vi "GetStartingMainViReference.vi"(8 "error in (no error)":errorcluster caption="Fehler (Eingang, kein Fehler)", 11 "ApplicationInititialisation Eingang":refnum<class "ApplicationInititialisation.lvclass"> caption="DNL_LabVIEW Object in") -> (0 "error out":errorcluster caption="Fehler (Ausgang)", 1 "String":string, 2 "vi reference":refnum<vi>, 3 "ApplicationInititialisation Ausgang":refnum<class "ApplicationInititialisation.lvclass"> caption="DNL_LabVIEW Object out")   [LabVIEW 2013, in "ApplicationInititialisation.lvclass"]
uses:
  ApplicationInititialisation.lvclass
panel:
  out "Array":string[](array[string])
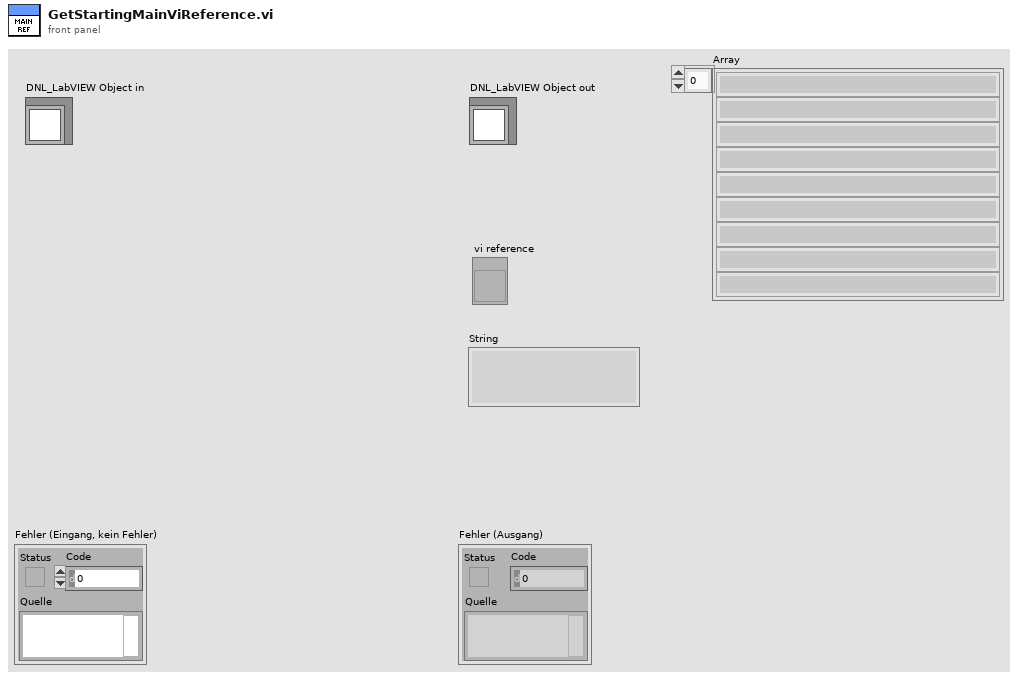
[diagram p1: front panel]
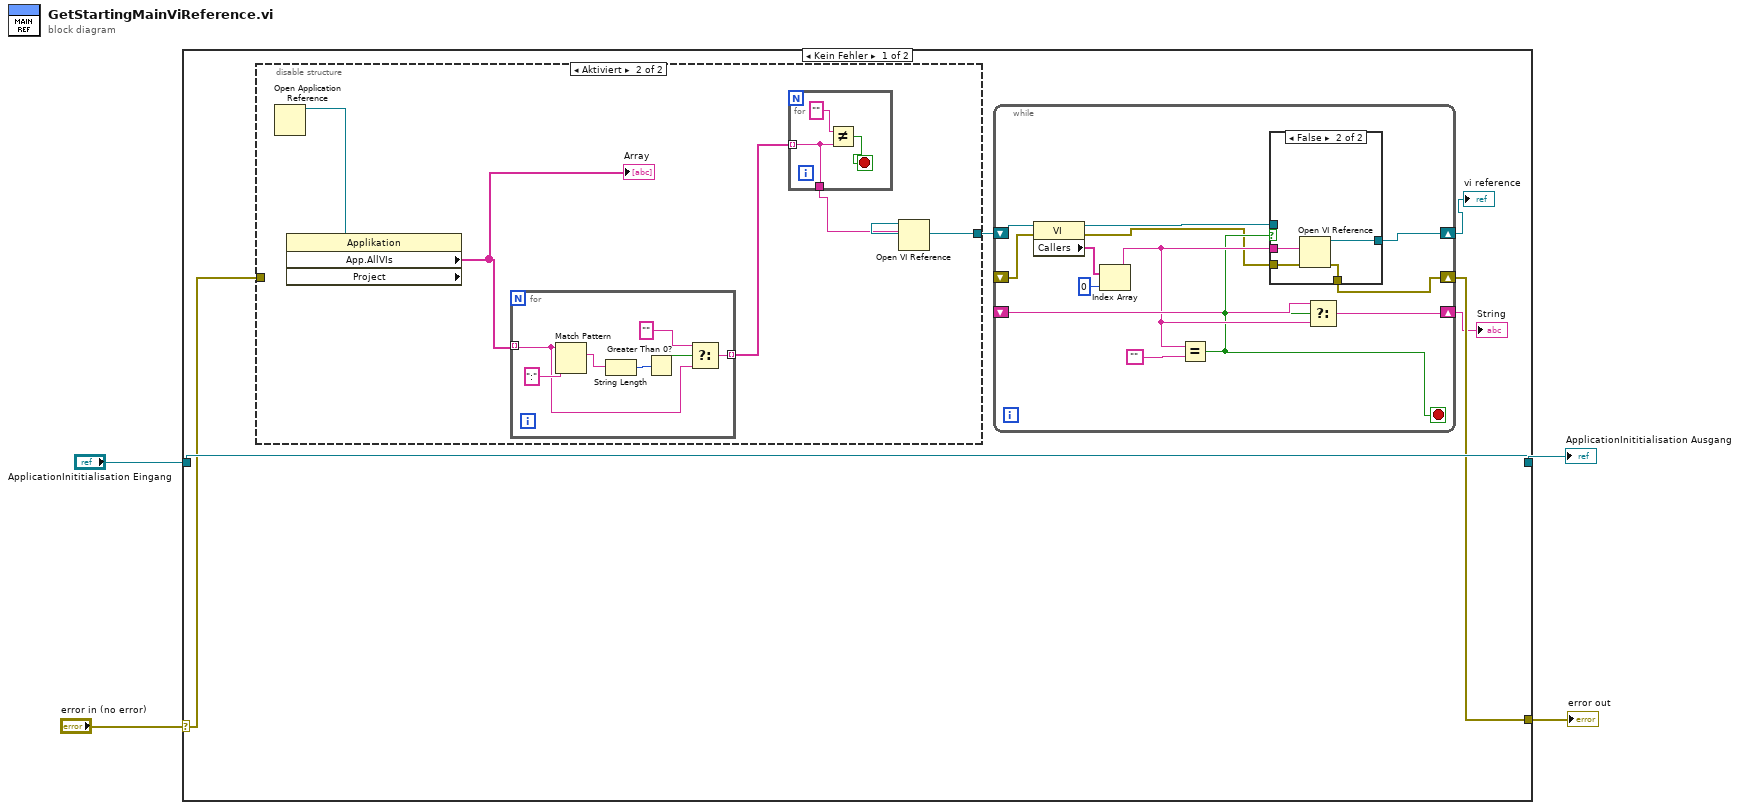
[diagram p0: block diagram]
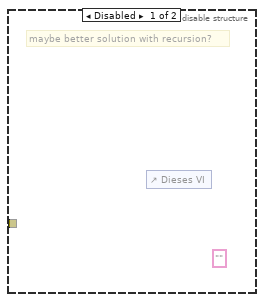
[diagram p3: hidden frame]
diagram:
  n1 = case shown="Kein Fehler" "error in (no error)" {
    selector: "error in (no error)" -> [w9 w47]
    tunnel: [w10 w48] -> w2
    tunnel: "ApplicationInititialisation Eingang" -> [w10 w48]
    tunnel: [w6 w47] -> w1
    frame No Error {
      n2 = disable-structure shown="Aktiviert" {
        disable-tunnel: [_ w35] -> w8
        disable-tunnel: w9 -> [w30 _]
        frame Disabled {
          (unwired) ""
          # "maybe better solution with recursion?"
          n3 = control-ref of="Dieses VI"() -> (w31:refnum<vi>)
        }
        frame Enabled {
          n4 = Open Application Reference() -> (3:w36:refnum<vi>)  [unwired: 4 in, 1 out]
          n5 = property class="Applikation" props=["App.AllVIs", "Project"](reference=w36) -> ("App.AllVIs"=w32:string[])  [unwired: 1 in, 3 out]
          "Array" <- w32
          n6 = for {
            tunnel: w32 -> [w41] mode=indexing
            tunnel: [w40] -> w34 mode=indexing
            n7 = Match Pattern(string=w41, regular expression=":" ("Format-String")) -> (match substring=w43:string)  [unwired: 1 in, 3 out]
            n8 = String Length(string=w43) -> (length=w45:i32)
            n9 = Greater Than 0?(x=w45) -> (x > 0?=w44:bool)
            n10 = Select(t="", s=w44, f=w41) -> (s? t:f=w40:string)
          }
          n11 = for {
            tunnel: w34 -> [w37] mode=indexing
            tunnel: [w37] -> w33
            stop <- w38 stop-if-true
            n12 = Not Equal?(x="" ("t"), y=w37) -> (x != y?=w38:bool)
          }
          n13 = Open VI Reference(vi path=w33) -> (vi reference=w35:refnum<vi>)  [unwired: 5 in, 1 out]
        }
      }
      n14 = while {
        shift-right: [w20] -> w7
        shift-left: w8 -> [w21]
        shift-right: [w16] -> w5
        shift-left: _ -> [w18]
        shift-right: [w11] -> w6
        shift-left: _ -> [w13]
        stop <- w14 stop-if-true
        n15 = property class="VI"(reference=w21, error in=w13) -> (reference out=w15:refnum<vi>, error out=w12:errorcluster, "Callers"=w22:string[])
        n16 = Index Array(array=w22, index=0 ("Index")) -> (element=w17:string)
        n17 = Equal?(x=w17, y="") -> (x = y?=w14:bool)
        n18 = case shown="False" w14 {
          tunnel: [w25 w29] -> w20
          tunnel: w17 -> [_ w28]
          tunnel: w15 -> [w25 _]
          tunnel: w12 -> [w24 w27]
          tunnel: [w24 w26] -> w11
          frame True {
          }
          frame False {
            n19 = Open VI Reference(vi path=w28, error in (no error)=w27) -> (vi reference=w29:refnum<vi>, error out=w26:errorcluster)  [unwired: 4 in]
          }
        }
        n20 = Select(t=w18, s=w14, f=w17) -> (s? t:f=w16:string)
      }
      "vi reference" <- w7
      "String" <- w5
    }
    frame Error {
    }
  }
  "error out" <- w1
  "ApplicationInititialisation Ausgang" <- w2
